vi "RUSHShooterPrimed.vi"(0 "IndexerSpeed":dbl, 5 "WheelSpeedF":dbl, 7 "WheelSpeedB":dbl, 9 "ShootStartWheels":bool, 11 "ShootIndexerEnable":bool) -> (4 "ShootOutIndexer":dbl, 6 "ShootOutWheelB":dbl, 8 "ShootOutWheelF":dbl)   [LabVIEW 2012]
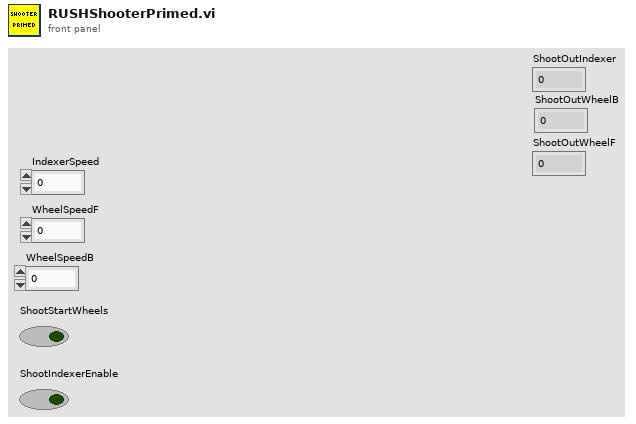
[diagram p1: front panel]
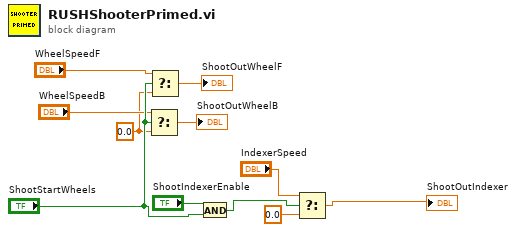
[diagram p0: block diagram]
diagram:
  w1 = 0.0 ("f")
  n1 = Select(t="WheelSpeedB", s="ShootStartWheels", f=w1) -> (s? t:f=→"ShootOutWheelB":dbl)
  n2 = Select(t="WheelSpeedF", s="ShootStartWheels", f=w1) -> (s? t:f=→"ShootOutWheelF":dbl)
  n3 = And(x="ShootIndexerEnable", y="ShootStartWheels") -> (x .and. y?=w7:bool)
  n4 = Select(t="IndexerSpeed", s=w7, f=0.0) -> (s? t:f=→"ShootOutIndexer":dbl)
